vi "Get_Max_Voltage.vi"(8 "error in":errorcluster, 11 "VISA name":refnum<visa-resource-name>) -> (0 "error out":errorcluster, 1 "valid":bool, 2 "max Voltage /V":dbl, 3 "VISA out":refnum<visa-resource-name>)   [LabVIEW 2020]
panel:
  out "read buffer":string
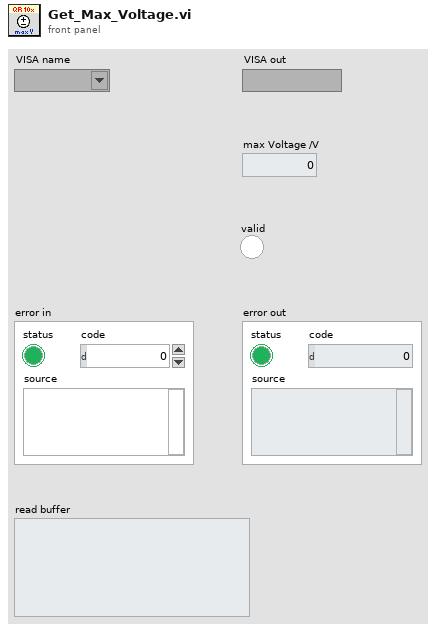
[diagram p1: front panel]
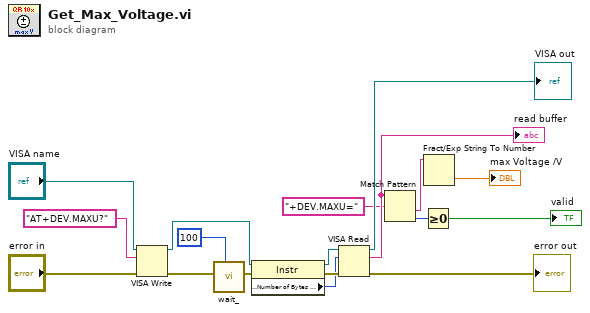
[diagram p0: block diagram]
diagram:
  n1 = VISA Write(VISA resource name="VISA name", write buffer="AT+DEV.MAXU?", error in (no error)="error in") -> (VISA resource name out=w14:refnum<visa-resource-name>, error out=w3:errorcluster)  [unwired: 1 out]
  n2 = call <instrlib>:"wait_.vi"("milliseconds to wait"=u32 100, "error in"=w3) -> ("error out"=w2:errorcluster)  [unwired: 9 in]
  n3 = property class="Instr"(reference=w14, error in=w2) -> (reference out=w10:refnum<visa-resource-name>, error out=w12:errorcluster, "Serial Settings:Number of Bytes at Serial Port"=w11:u32)
  n4 = VISA Read(VISA resource name=w10, byte count=w11, error in (no error)=w12) -> (VISA resource name out=→"VISA out":refnum<visa-resource-name>, read buffer=w9:string, error out=→"error out":errorcluster)  [unwired: 1 out]
  "read buffer" <- w9
  n5 = Match Pattern(string=w9, regular expression="+DEV.MAXU=") -> (after substring=w7:string, offset past match=w5:i32)  [unwired: 1 in, 2 out]
  n6 = Greater Or Equal To 0?(x=w5) -> (x >= 0?=→"valid":bool)
  n7 = Fract/Exp String To Number(string=w7) -> (number=→"max Voltage /V":dbl)  [unwired: 3 in, 1 out]
